vi "SampleHTIRSeekerV2.vi"   [LabVIEW 2009]
uses:
  <vilib>/NXT/HiTechnic/subVIs/HiTechnic Port.ctl
  <vilib>/NXT/Block Support/NXT_InputPort.ctl
  <vilib>/NXT/Dual Mode Library/Display/drawText.vi
types:
  T1 = typedef "LVHSConnector.ctl" = cluster{"error":errorcluster, "address":string, "NXT #":i32, "Show Error":bool, "Connection":u16}
  T2 = typedef "HiTechnic Port.ctl" = cluster{"Port":T3, "MUX Port":u8}
  T3 = typedef "NXT_InputPort.ctl" = u8
  T4 = cluster{"Direction (0-9)":u8, "Signal Strength (Array)":u8[]}
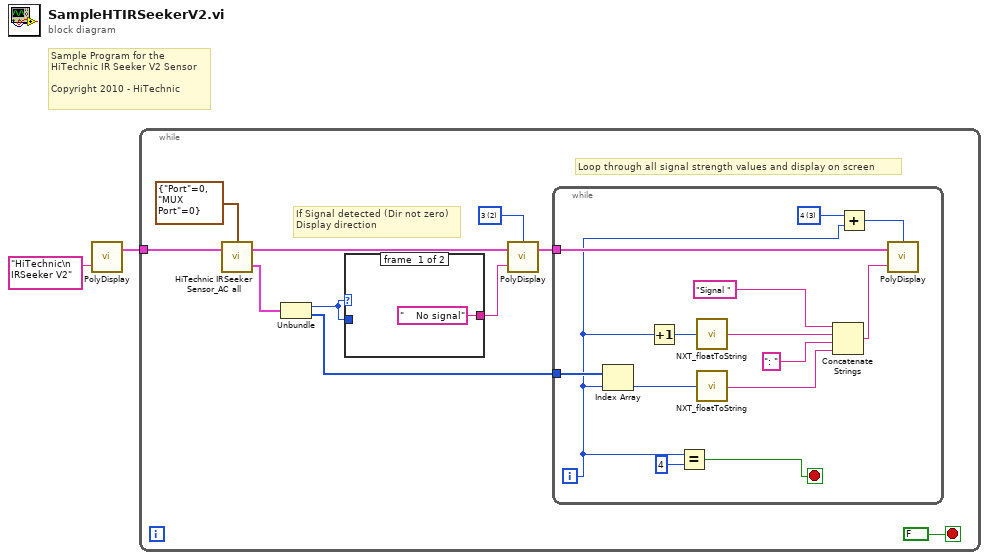
[diagram p0: block diagram]
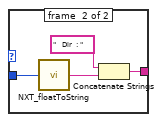
[diagram p2: hidden frame]
diagram:
  # "Sample Program for the\nHiTechnic IR Seeker V2 Sensor\n\nCopyright 2010 - HiTechnic"
  n1 = call-poly <vilib>:"PolyDisplay.vi"("Text"="HiTechnic\n  IRSeeker V2") -> ("NXT"=w2:T1)  [unwired: 3 in]
  n2 = while {
    tunnel: w2 -> [w8]
    stop <- FALSE stop-if-true
    w7 = i16 2 items=["1", "2", "3", "4", "5", "6", "7", "8"] ("Line")
    # "Loop through all signal strength values and display on screen"
    # "If Signal detected (Dir not zero)\nDisplay direction"
    n3 = call <vilib>:"HiTechnic IRSeeker Sensor_AC all.vi"("NXT"=w8, "Port/MUX"=T2 {"Port"=0, "MUX Port"=0}) -> ("All Info"=w12:T4, "NXT"=w11:T1)  [unwired: 1 in]
    n4 = Unbundle(w12) -> ("Direction (0-9)"=w3:u8, "Signal Strength (Array)"=w10:u8[])
    n5 = case shown="0" w3 {
      tunnel: w3 -> [_ w17]
      tunnel: ["    No signal" w14] -> w9
      frame #0 {
      }
      frame #1 {
        n6 = call <vilib>:"NXT_floatToString.vi"("number"=w17) -> ("string"=w15:string)
        n7 = Concatenate Strings("   Dir  : " ("string"), w15) -> (w14:string)
      }
    }
    n8 = call-poly <vilib>:"PolyDisplay.vi"("Text"=w9, "NXT"=w11, "Line"=w7) -> ("NXT"=w6:T1)  [unwired: 1 in]
    n9 = while {
      tunnel: w10 -> [w31]
      tunnel: w6 -> [w20]
      i -> [w18]
      stop <- w30 stop-if-true
      w22 = i16 3 items=["1", "2", "3", "4", "5", "6", "7", "8"] ("Line")
      n10 = Index Array(array=w31, index=w18) -> (element=w27:u8)
      n11 = Increment(x=w18) -> (x+1=w28:i32)
      n12 = Equal?(x=w18, y=4) -> (x = y?=w30:bool)
      n13 = call <vilib>:"NXT_floatToString.vi"("number"=w28) -> ("string"=w25:string)
      n14 = call <vilib>:"NXT_floatToString.vi"("number"=w27) -> ("string"=w23:string)
      n15 = Concatenate Strings("Signal " ("string"), w25, ": " ("string"), w23) -> (w19:string)
      n16 = Add(x=w22, y=w18) -> (x+y=w21:i32)
      n17 = call-poly <vilib>:"PolyDisplay.vi"("Text"=w19, "NXT"=w20, "Line"=w21) -> ()  [unwired: 1 in, 1 out]
    }
  }
